vi "Teleop.vi"(10 "Match Info":T1={"Autonomous Elapsed Seconds"=0.0, "TeleOp Elapsed Seconds"=0.0, "Disabled Elapsed Seconds"=0.0, "Visited Autonomous"=FALSE, "Visited TeleOp"=FALSE, "Visited Disabled"=FALSE, "Autonomous Settings"={"Autonomous Style"=enum."Independent", "VI Refnum"=refnum}}, 11 "Call Context":T2) -> ()   [LabVIEW 2019]
doc: "This VI is called for each enabled TeleOp packet received from the DS. It is typically used to read from joysticks and other inputs and update I/O or setpoints for timed control loops. It should complete and return within 20 milliseconds or risk missing DS packets."
uses:
  <vilib>/Rock Robotics/WPI/DriverStation/WPI_DriverStationDerivedRobotMode.ctl
  <vilib>/Rock Robotics/WPI/DriverStation/WPI_DriverStationMatch Info.ctl
  <vilib>/Rock Robotics/WPI/Utilities/WPI_GetSetVariantRefNum.vi
  <vilib>/Rock Robotics/Network Tables/NT Write Boolean Array.vi
  <vilib>/Rock Robotics/Network Tables/NT Write Numeric Array.vi
  <vilib>/Rock Robotics/WPI/DriverStation/WPI_DriverStationRobotMode2.ctl
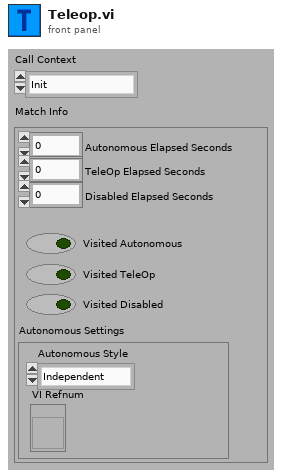
[diagram p1: front panel]
types:
  T1 = typedef "WPI_DriverStationMatch Info.ctl" = cluster{"Autonomous Elapsed Seconds":dbl, "TeleOp Elapsed Seconds":dbl, "Disabled Elapsed Seconds":dbl, "Visited Autonomous":bool, "Visited TeleOp":bool, "Visited Disabled":bool, "Autonomous Settings":cluster{"Autonomous Style":enum16{"Iterative", "Independent"}, "VI Refnum":refnum<vi>}}
  T2 = typedef "WPI_DriverStationDerivedRobotMode.ctl" = enum16{"Init", "Execute", "Stop"}
  T3 = typedef "WPI_JoystickDevRef.ctl" = cluster{"Device":T4}
  T4 = typedef "WPI_JoystickDeviceEnum.ctl" = enum16{"USB 0", "USB 1", "USB 2", "USB 3", "USB 4", "USB 5"}
  T5 = typedef "WPI_DriverStationRobotMode2.ctl" = enum16{"Autonomous Disabled", "Autonomous Enabled", "Teleop Disabled", "Teleop Enabled", "Disconnected", "Finish", "Test Disabled", "Test Enabled", "Emergency Stopped"}
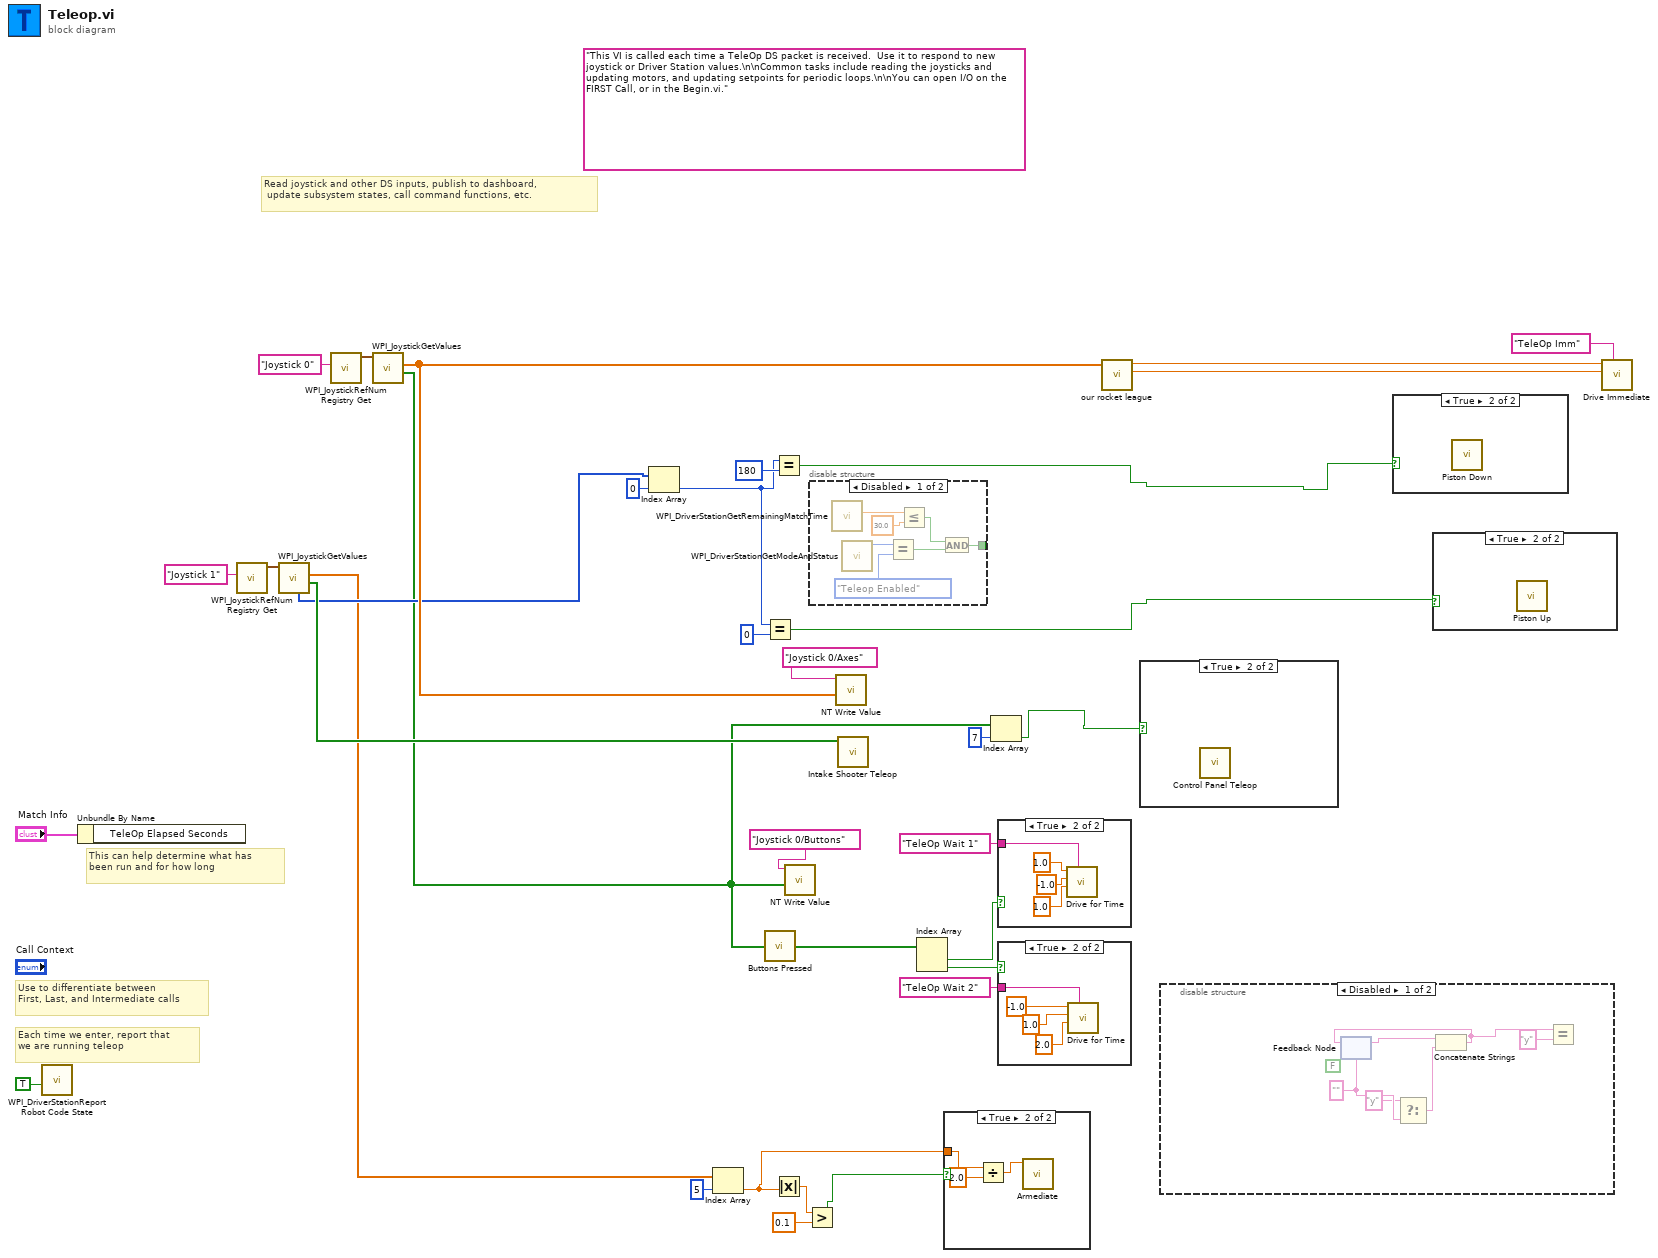
[diagram p0: block diagram]
diagram:
  (unwired) "This VI is called each time a TeleOp DS packet is received.  Use it to respond to new joystick or Driver Station values.\n\nCommon tasks include reading the joysticks and updating motors, and updating setpoints for periodic loops.\n\nYou can open I/O on the FIRST Call, or in the Begin.vi."
  # "Read joystick and other DS inputs, publish to dashboard,\n update subsystem states, call command functions, etc."
  # "Each time we enter, report that\nwe are running teleop"
  # "Use to differentiate between\nFirst, Last, and Intermediate calls"
  # "This can help determine what has\nbeen run and for how long"
  n1 = call <vilib>:"WPI_DriverStationReport Robot Code State.vi"("TeleOp"=TRUE ("Autonomous")) -> ()  [unwired: 10 in, 1 out]
  n2 = Unbundle By Name("Match Info") -> ()  [unwired: 1 out]
  n3 = call <vilib>:"WPI_JoystickRefNum Registry Get.vi"("refnum name"="Joystick 1") -> ("JoystickDevRef"=w18:T3)  [unwired: 1 in, 9 out]
  n4 = call <vilib>:"WPI_JoystickGetValues.vi"("JoystickDevRef"=w18) -> ("Buttons"=w17:bool[], "Axes"=w15:dbl[], "POVs"=w16:i16[])  [unwired: 6 in, 2 out]
  n5 = call <vilib>:"WPI_JoystickRefNum Registry Get.vi"("refnum name"="Joystick 0") -> ("JoystickDevRef"=w31:T3)  [unwired: 1 in, 9 out]
  n6 = call <vilib>:"WPI_JoystickGetValues.vi"("JoystickDevRef"=w31) -> ("Buttons"=w3:bool[], "Axes"=w24:dbl[])  [unwired: 6 in, 3 out]
  n7 = Index Array(array=w16, index=0) -> (element=w6:i16)
  n8 = Index Array(array=w15, index=5) -> (element=w10:dbl)
  n9 = Equal?(x=w6, y=i16 0) -> (x = y?=w5:bool)
  n10 = call "Buttons Pressed.vi"("Button Values"=w3) -> ("Button Presses"=w23:bool[])
  n11 = Equal?(x=w6, y=i16 180) -> (x = y?=w4:bool)
  n12 = Absolute Value(x=w10) -> (abs(x)=w14:dbl)
  n13 = call-poly <vilib>:"NT Write Value.vi"("Boolean Array"=w3, "Name"="Joystick 0/Buttons") -> ()  [unwired: 9 in, 1 out]
  n14 = Greater?(x=w14, y=0.1) -> (0:w12:bool)
  n15 = disable-structure shown="Disabled" {
    disable-tunnel: [w35 _] -> _
    frame Disabled {
      n16 = call <vilib>:"WPI_DriverStationGetRemainingMatchTime.vi"() -> ("Match Time(s)"=w39:sgl)  [unwired: 10 in, 1 out]
      n17 = call <vilib>:"WPI_DriverStationGetModeAndStatus.vi"() -> ("Robot Mode"=w41:T5)  [unwired: 10 in, 1 out]
      n18 = Equal?(x=w41, y=WPI_DriverStationRobotMode2."Teleop Enabled") -> (x = y?=w36:bool)
      n19 = Less Or Equal?(x=w39, y=sgl 30.0) -> (x <= y?=w37:bool)
      n20 = And(x=w37, y=w36) -> (x .and. y?=w35:bool)
    }
    frame Enabled {
    }
  }
  n21 = call-poly <vilib>:"NT Write Value.vi"("Numeric Array"=w24, "Name"="Joystick 0/Axes") -> ()  [unwired: 9 in, 1 out]
  n22 = call "Intake Shooter Teleop.vi"("Buttons"=w17) -> ()  [unwired: 11 in]
  n23 = Index Array(array=w23) -> (element #1=w28:bool, element #2=w27:bool)  [unwired: 2 in]
  n24 = case shown="True" w12 {
    tunnel: w10 -> [_ w44]
    frame False {
    }
    frame True {
      n25 = Divide(x=w44, y=2.0) -> (x/y=w42:dbl)
      n26 = call "Armediate.vi"("Setpoint"=w42) -> ()  [unwired: 10 in, 1 out]
    }
  }
  n27 = Index Array(array=w3, index=7) -> (element=w1:bool)
  n28 = case shown="True" w28 {
    tunnel: "TeleOp Wait 1" ("Description") -> [_ w47]
    frame False {
    }
    frame True {
      n29 = call "Drive for Time.vi"("Description"=w47, "Seconds"=1.0, "Right Speed"=-1.0, "Left Speed"=1.0) -> ()  [unwired: 7 in, 1 out]
    }
  }
  n30 = case shown="True" w27 {
    tunnel: "TeleOp Wait 2" ("Description") -> [_ w50]
    frame False {
    }
    frame True {
      n31 = call "Drive for Time.vi"("Description"=w50, "Seconds"=2.0, "Right Speed"=1.0, "Left Speed"=-1.0) -> ()  [unwired: 7 in, 1 out]
    }
  }
  n32 = call "our rocket league.vi"("Axes"=w24) -> ("upper limit 2"=w20:dbl, "upper limit 3"=w21:dbl)  [unwired: 8 in, 1 out]
  n33 = case shown="True" w1 {
    frame False {
    }
    frame True {
      n34 = call "Control Panel Teleop.vi"() -> ()  [unwired: 12 in]
    }
  }
  n35 = disable-structure shown="Disabled" {
    frame Disabled {
      w54 = FALSE
      w59 = ""
      n36 = feedback #1(w59) -> (w60:string)
      n37 = Select(t="y", f=w59) -> (s=w53:bool, s? t:f=w58:string)
      n38 = Concatenate Strings(w60, w58) -> (w56:string)
      n39 = feedback-in #1(w56) -> ()
      n40 = Equal?(x=w56, y="y") -> ()  [unwired: 1 out]
    }
    frame Enabled {
    }
  }
  n41 = case shown="True" w4 {
    frame False {
    }
    frame True {
      n42 = call "Piston Down.vi"() -> ()  [unwired: 11 in, 1 out]
    }
  }
  n43 = case shown="True" w5 {
    frame False {
    }
    frame True {
      n44 = call "Piston Up.vi"() -> ()  [unwired: 11 in, 1 out]
    }
  }
  n45 = call "Drive Immediate.vi"("Description"="TeleOp Imm", "Right Setpoint"=w20, "Left Setpoint"=w21) -> ()  [unwired: 8 in, 1 out]
